vi "niusrprios Generate Waveform.vi"   [LabVIEW 2015]
doc: "Creates a waveform to send to a device for generation."
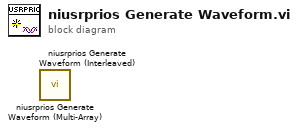
[diagram p0: block diagram]
diagram:
  n1 = call "niusrprios Generate Waveform (Multi-Array).vi"() -> ()  [unwired: 12 in, 4 out]
  n2 = call "niusrprios Generate Waveform (Interleaved).vi"() -> ()  [unwired: 13 in, 3 out]
